vi "XMLOpenConfiguration.vi"(8 "Error In":errorcluster, 11 "path to XML document":path) -> (0 "Error Out":errorcluster, 2 "Parse Errors":string, 3 "DOM document out":refnum<k20>)   [LabVIEW 2014, in "OPCUA XML(dev).lvlib"]
uses:
  OPCUA XML(dev).lvlib
  <resource>/objmgr/DOMUserDefRef.rc
  <vilib>/xml/NI_XML.lvlib
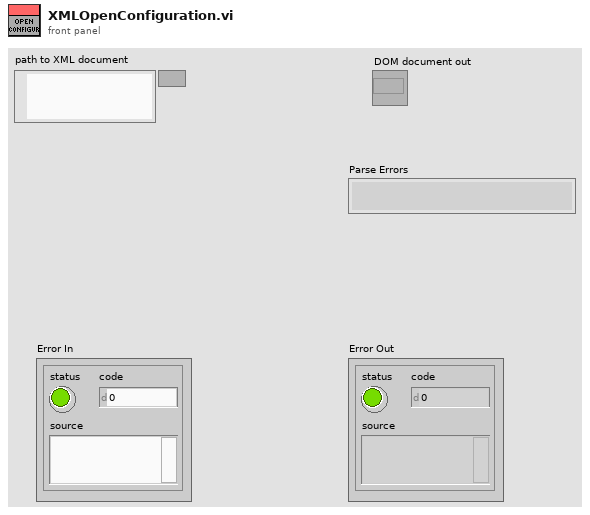
[diagram p1: front panel]
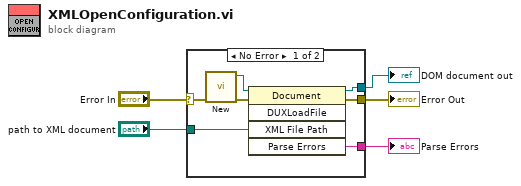
[diagram p0: block diagram]
diagram:
  n1 = case shown="No Error" "Error In" {
    selector: "Error In" -> [w8 w13]
    tunnel: [w9 w13] -> w5
    tunnel: "path to XML document" -> [w10 _]
    tunnel: [w7 _] -> w2
    tunnel: [w6 _] -> w1
    frame No Error {
      n2 = call <vilib>:"New.vi"("error in (no error)"=w8) -> ("error out"=w12:errorcluster, "DOM document out"=w11:refnum<k20>)  [unwired: 7 out]
      n3 = invoke class="Document" method="DUXLoadFile"(reference=w11, error in=w12, "XML File Path"=w10) -> (reference out=w7:refnum<k20>, error out=w9:errorcluster, "Parse Errors"=w6:string)  [unwired: 2 in, 2 out]
    }
    frame Error {
    }
  }
  "Error Out" <- w5
  "DOM document out" <- w2
  "Parse Errors" <- w1
